vi "get sonde data.vi"(8 "error in (no error)":errorcluster, 11 "Sonde Output File Path":path) -> (0 "error out":errorcluster, 1 "Sample Row \nBreak points":i32[](array[numeric]), 2 "Sample Array":i32[](array[numeric]), 3 "Sonde Data":string[][](array[string]))   [LabVIEW 2016]
uses:
  <vilib>/Utility/file.llb/Read Delimited Spreadsheet (string).vi
panel:
  out "Sample column":string[](array[string])
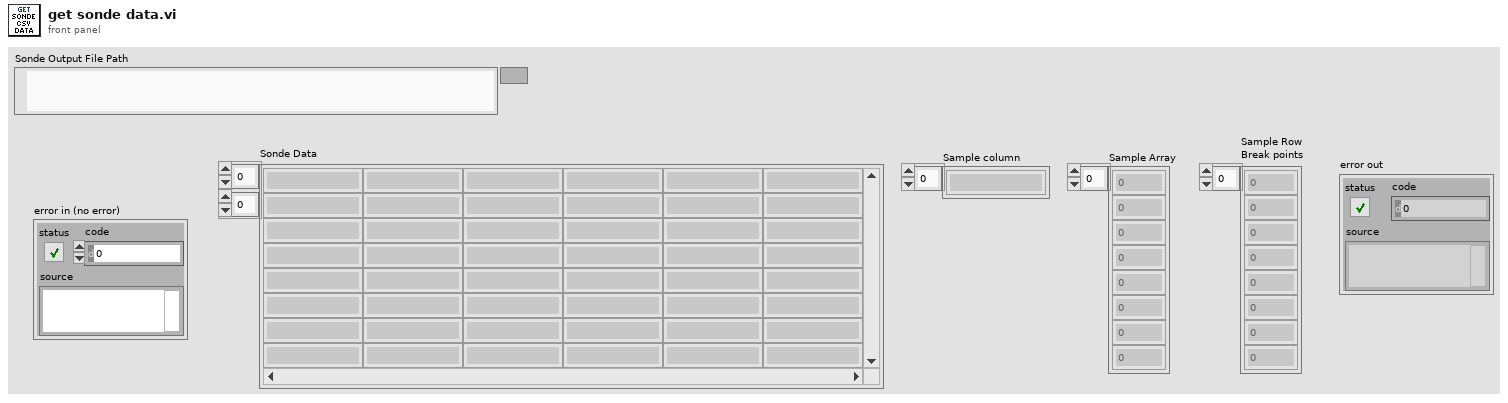
[diagram p1: front panel]
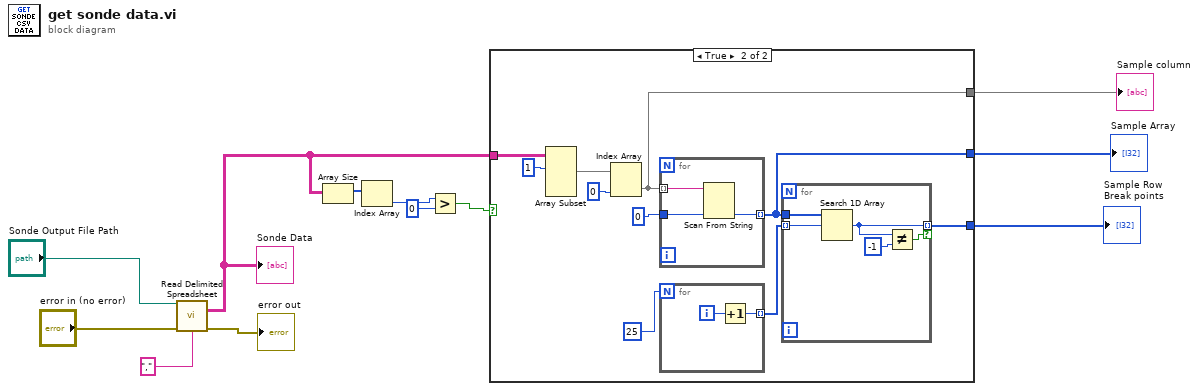
[diagram p0: block diagram]
diagram:
  n1 = call-poly <vilib>:"Read Delimited Spreadsheet.vi"("file path (dialog if empty)"="Sonde Output File Path", "error in (no error)"="error in (no error)", "delimiter (\\t)"="," ("delimiter (\\t)")) -> ("all rows"=w5:string[][], "error out"=→"error out":errorcluster)  [unwired: 7 in, 4 out]
  "Sonde Data" <- w5
  n2 = Array Size(array=w5) -> (size(s)=w4:i32[])
  n3 = Index Array(array=w4) -> (element=w3:i32)  [unwired: 1 in]
  n4 = Greater?(x=w3, y=0) -> (0:w1:bool)
  n5 = case shown="True" w1 {
    tunnel: w5 -> [_ w21]
    tunnel: [_ w18] -> w8
    tunnel: [_ w16] -> w7
    tunnel: [_ w13] -> w6
    frame False {
    }
    frame True {
      n6 = Array Subset(array=w21, index (row)=1 ("index")) -> (w19:string[][])  [unwired: 3 in]
      n7 = Index Array(array=w19, index (col)=0 ("disabled index (col)")) -> (element=w18:string[])  [unwired: 1 in]
      n8 = for {
        tunnel: w18 -> [w32] mode=indexing
        tunnel: 0 -> [w31]
        tunnel: [w30] -> w16 mode=indexing
        n9 = Scan From String(input string=w32, default 1=w31) -> (output 1=w30:i32)  [unwired: 3 in, 3 out]
      }
      n10 = for {
        N: 25 -> [_]
        tunnel: [w23] -> w14 mode=indexing
        i -> [w24]
        n11 = Increment(x=w24) -> (x+1=w23:i32)
      }
      n12 = for {
        tunnel: w16 -> [w29]
        tunnel: w14 -> [w28] mode=indexing
        tunnel: [w27] -> w13 mode=indexing if=w25
        n13 = Search 1D Array(1D array=w29, element=w28) -> (index of element=w27:i32)  [unwired: 1 in]
        n14 = Not Equal?(x=w27, y=-1) -> (x != y?=w25:bool)
      }
    }
  }
  "Sample column" <- w8
  "Sample Array" <- w7
  "Sample Row \nBreak points" <- w6
